vi "SWLDA_constructor.vi"() -> ()   [LabVIEW 2014]
uses:
  <vilib>/Utility/file.llb/Read From Spreadsheet File (string).vi
  <vilib>/Utility/file.llb/Read From Spreadsheet File (I64).vi
panel:
  in  "discard_channel":path
  in  "Training Path":path
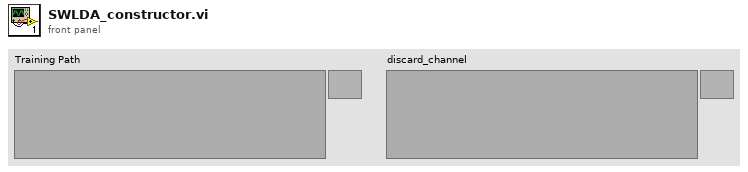
[diagram p1: front panel]
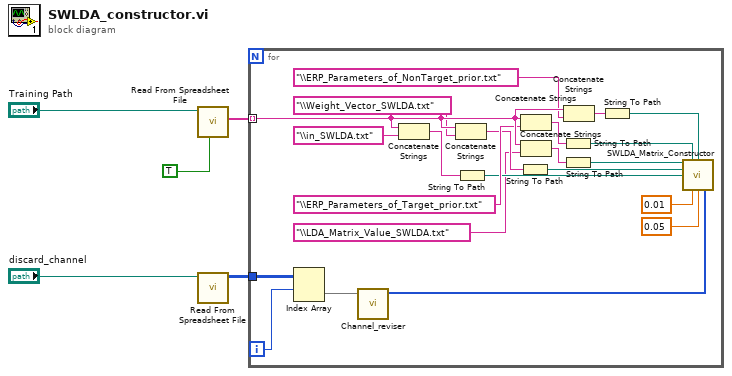
[diagram p0: block diagram]
diagram:
  n1 = call-poly <vilib>:"Read From Spreadsheet File.vi"("transpose (no:F)"=TRUE, "file path (dialog if empty)"="Training Path") -> ("first row"=w3:string[])  [unwired: 5 in, 4 out]
  n2 = call-poly <vilib>:"Read From Spreadsheet File.vi"("file path (dialog if empty)"="discard_channel") -> ("all rows"=w1:i64[][])  [unwired: 6 in, 4 out]
  n3 = for {
    tunnel: w3 -> [w27] mode=indexing
    tunnel: w1 -> [w9]
    i -> [w8]
    n4 = Index Array(array=w9, index (row)=w8) -> (element=w7:i64[])  [unwired: 1 in]
    n5 = call "Channel_reviser.vi"("CHANNEL_ARRAY"=w7) -> ("CHANNEL_ARRAY_revised"=w6:i64[])  [unwired: 10 in]
    n6 = Concatenate Strings(w27, "\\in_SWLDA.txt" ("string")) -> (w17:string)
    n7 = Concatenate Strings(w27, "\\Weight_Vector_SWLDA.txt" ("string")) -> (w18:string)
    n8 = String To Path(string=w17) -> (path=w15:path)
    n9 = String To Path(string=w18) -> (path=w16:path)
    n10 = Concatenate Strings(w27, "\\ERP_Parameters_of_Target_prior.txt") -> (w23:string)
    n11 = Concatenate Strings(w27, "\\LDA_Matrix_Value_SWLDA.txt" ("string")) -> (w20:string)
    n12 = String To Path(string=w23) -> (path=w21:path)
    n13 = String To Path(string=w20) -> (path=w19:path)
    n14 = Concatenate Strings(w27, "\\ERP_Parameters_of_NonTarget_prior.txt") -> (w24:string)
    n15 = String To Path(string=w24) -> (path=w22:path)
    n16 = call "SWLDA_Matrix_Constructor.vi"("SWLDA_Matrix"=w19, "ERP_Target"=w21, "ERP_Nontarget"=w22, "Weight_SWLDA"=w16, "in"=w15, "penter"=0.01, "premove"=0.05 ("penter"), "DIscard Channel Info"=w6) -> ()  [unwired: 8 in]
  }
